vi "Errorin loop.vi"() -> ()   [LabVIEW 2022 SP3]
uses:
  <vilib>/Utility/error.llb/DialogType.ctl
panel:
  out "text":string
  in  "Path":path
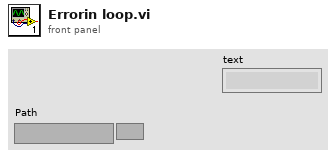
[diagram p1: front panel]
types:
  T1 = typedef "DialogType.ctl" = u16
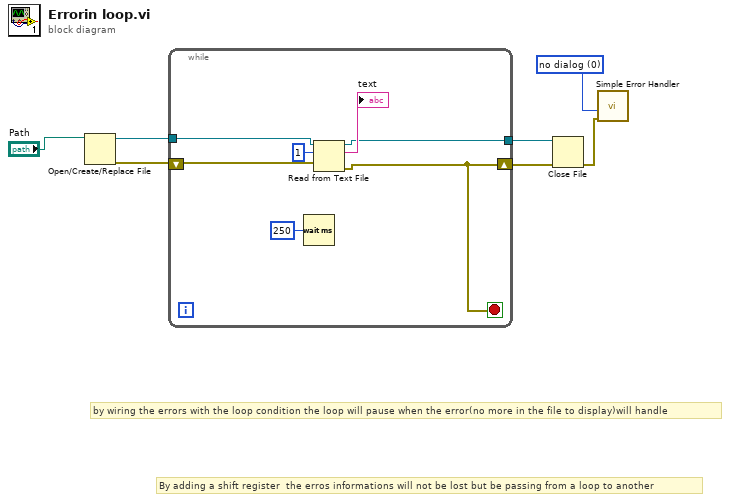
[diagram p0: block diagram]
diagram:
  w1 = T1 0 items=["no dialog", "OK message", "continue or stop message", "OK message + warnings", "continue/stop + warnings"] ("type of dialog (OK msg:1)")
  # "By adding a shift register  the erros informations will not be lost but be passing from a loop to another"
  # "by wiring the errors with the loop condition the loop will pause when the error(no more in the file to display)will handle"
  n1 = Open/Create/Replace File(file path (use dialog)="Path") -> (refnum out=w6:refnum<file>, error out=w5:errorcluster)  [unwired: 5 in, 1 out]
  n2 = while {
    tunnel: w6 -> [w14]
    tunnel: [w9] -> w3
    shift-right: [w8] -> w4
    shift-left: w5 -> [w13]
    stop <- w8 stop-if-true
    n3 = Wait (ms)(milliseconds to wait=u32 250) -> ()  [unwired: 1 out]
    n4 = Read from Text File(file (use dialog)=w14, count=1, error in=w13) -> (refnum out=w9:refnum<file>, text=→"text":string, error out=w8:errorcluster)  [unwired: 1 in, 1 out]
  }
  n5 = Close File(refnum=w3, error in=w4) -> (error out=w2:errorcluster)  [unwired: 1 out]
  n6 = call <vilib>:"Simple Error Handler.vi"("type of dialog (OK msg:1)"=w1, "error in (no error)"=w2) -> ()  [unwired: 3 in, 5 out]
